vi "InicializarContador.vi"(2 "stop 2":refnum<vi>, 9 "WreadInicio":refnum<vi>) -> ()   [LabVIEW 2010]
panel:
  in  "Inicio":i32
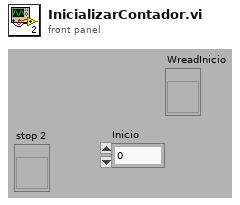
[diagram p1: front panel]
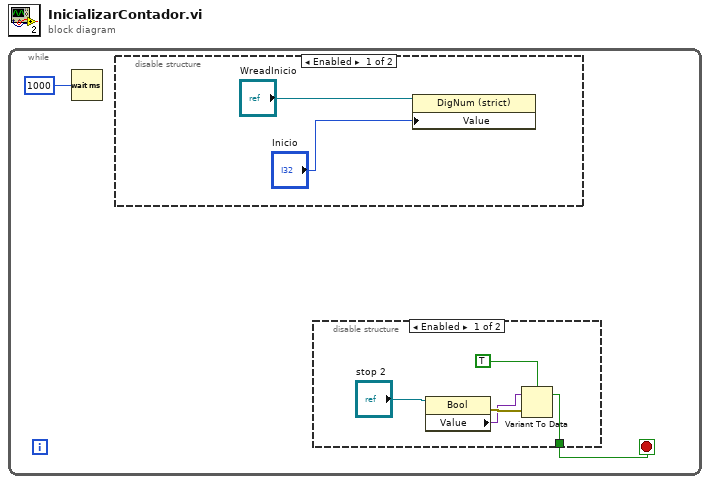
[diagram p0: block diagram]
diagram:
  n1 = while {
    stop <- w1 stop-if-true
    n2 = Wait (ms)(milliseconds to wait=u32 1000) -> ()  [unwired: 1 out]
    n3 = disable-structure shown="Enabled" {
      frame Enabled {
        n4 = property class="DigNum (strict)"(reference="WreadInicio", "Value"="Inicio") -> ()  [unwired: 1 in, 2 out]
      }
      frame Disabled {
      }
    }
    n5 = disable-structure shown="Enabled" {
      disable-tunnel: [w6 _] -> w1
      frame Enabled {
        n6 = property class="Bool"(reference="stop 2") -> (error out=w8:errorcluster, "Value"=w7:variant)  [unwired: 1 in, 1 out]
        n7 = Variant To Data(error in=w8, Variant=w7, type=TRUE) -> (data=w6:bool)  [unwired: 1 out]
      }
      frame Disabled {
      }
    }
  }
